vi "combo.vi"() -> ()   [LabVIEW 2018]
panel:
  in  "Tab Control":T1(tab)
  out "discharge for \ncapacitor":dbl
  in  "t":dbl
  in  "c":dbl
  in  "R":dbl
  in  "Vo":dbl
  in  "E":dbl
  out "Vl angle":dbl
  out "Vl":dbl
  out "Vr angle":dbl
  out "Vr":dbl
  out "I angle":dbl
  out "I":dbl
  out "Zt angle":dbl
  out "Zt":dbl
  in  "L1":dbl
  in  "C1":dbl
  in  "R1":dbl
  in  "V1 angle":dbl
  in  "V1":dbl
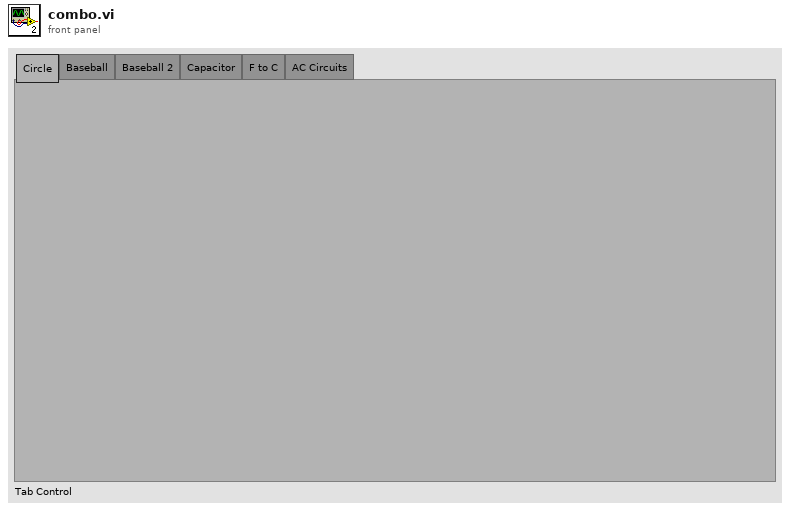
[diagram p1: front panel]
types:
  T1 = enum32{"Circle", "Baseball", "Baseball 2", "Capacitor", "F to C", "AC Circuits"}
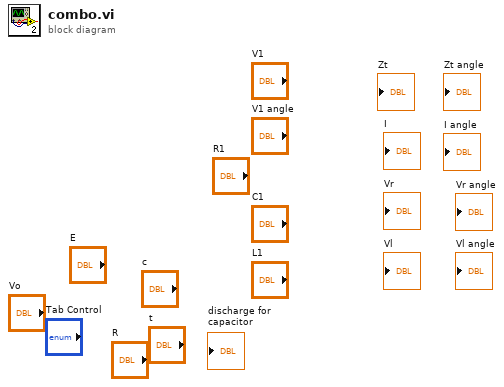
[diagram p0: block diagram]
diagram:
